vi "Labspec GetMotorStatus.vi"(7 "error in":errorcluster, 8 "Motor Name":T1=enum."Hole", 9 "MotorID":i32, 10 "Automation Refnum In":refnum<k7>) -> (0 "error out":errorcluster, 2 "Ready?":bool, 3 "Automation Refnum Out":refnum<k7>)   [LabVIEW 2014]
uses:
  MoveMotor Motor Name.ctl
panel:
  out "Motor Status":i16(ring) items=["Ready"=0, "Busy"=1, "Motor not present"=-1]
  # "LICENSED MATERIALS – PROPERTY OF IBM\nCopyright IBM Corp. 2016,\nALL RIGHTS RESERVED"
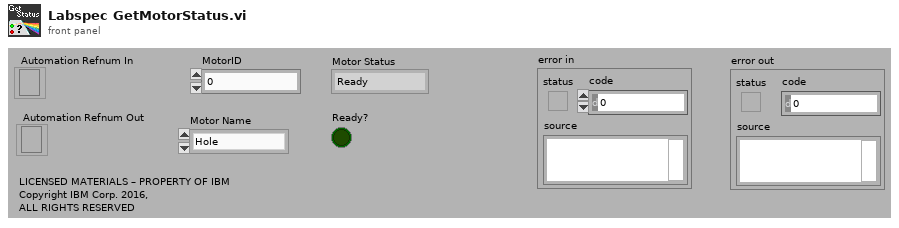
[diagram p1: front panel]
types:
  T1 = typedef "MoveMotor Motor Name.ctl" = enum16{"Spectro", "Premono", "Grating", "Slit", "Hole", "X", "Y", "XT", "YT", "XL", "YL", "Z", "Laser", "Filter", "Objective", "Detector", "Detector Temperature"}
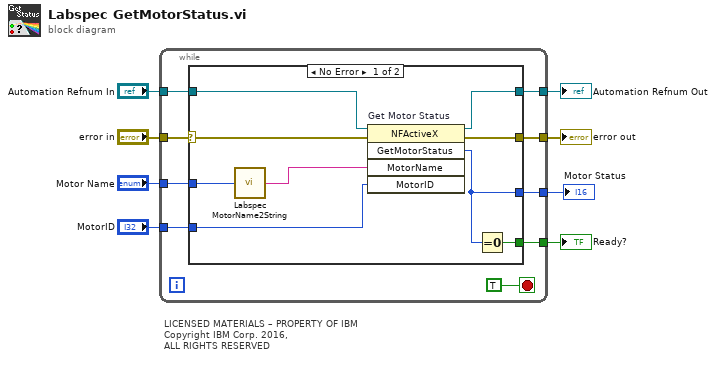
[diagram p0: block diagram]
diagram:
  # "LICENSED MATERIALS – PROPERTY OF IBM\nCopyright IBM Corp. 2016,\nALL RIGHTS RESERVED"
  n1 = while {
    tunnel: "Motor Name" -> [w17]
    tunnel: "Automation Refnum In" -> [w16]
    tunnel: [w15] -> w6
    tunnel: [w14] -> w5
    tunnel: "MotorID" -> [w13]
    tunnel: "error in" -> [w12]
    tunnel: [w11] -> w2
    tunnel: [w9] -> w1
    stop <- TRUE stop-if-true
    n2 = case shown="No Error" w12 {
      selector: w12 -> [w22 w27]
      tunnel: w17 -> [w19 _]
      tunnel: w16 -> [w26 w28]
      tunnel: [w25 w28] -> w15
      tunnel: [w24 w27] -> w14
      tunnel: w13 -> [w23 _]
      tunnel: [w21 _] -> w11
      tunnel: [w18 _] -> w9
      frame No Error {
        n3 = call "Labspec MotorName2String.vi"("Motor Name"=w19) -> ("PositionName"=w20:string)
        n4 = invoke on="Get Motor Status" class="NFActiveX" method="GetMotorStatus"(reference=w26, error in=w22, "MotorName"=w20, "MotorID"=w23) -> (reference out=w25:refnum<k7>, error out=w24:errorcluster, "GetMotorStatus"=w18:i32)  [unwired: 1 in, 2 out]
        n5 = Equal To 0?(x=w18) -> (x = 0?=w21:bool)
      }
      frame Error {
      }
    }
  }
  "error out" <- w5
  "Automation Refnum Out" <- w6
  "Ready?" <- w2
  "Motor Status" <- w1
